vi "data_waypoint_ref.vi"() -> ()   [LabVIEW 2018] (continued)
{"X"=175318.28403795866, "Y"=530191.9350482963}, {"X"=175318.32304521388, "Y"=530191.9869078569}, {"X"=175318.36204793068, "Y"=530192.0384311461}, {"X"=175318.4005898055, "Y"=530192.0898758835}, {"X"=175318.43864458468, "Y"=530192.1416494689}, {"X"=175318.47640338843, "Y"=530192.1930820906}, {"X"=175318.51419378835, "Y"=530192.2441161796}, {"X"=175318.55208232062, "Y"=530192.2944862834}, {"X"=175318.58985834898, "Y"=530192.3451530531}, {"X"=175318.62736532633, "Y"=530192.3949971002}, {"X"=175318.66480275526, "Y"=530192.4440855398}, {"X"=175318.70216220792, "Y"=530192.4937657638}, {"X"=175318.74007465132, "Y"=530192.5435342542}, {"X"=175318.77838922056, "Y"=530192.5935956714}, {"X"=175318.81680214155, "Y"=530192.6436667865}, {"X"=175318.85473180335, "Y"=530192.6944685044}, {"X"=175318.893105015, "Y"=530192.7454908877}, {"X"=175318.93198027203, "Y"=530192.7964474163}, {"X"=175318.97074562093, "Y"=530192.847981396}, {"X"=175319.00950281188, "Y"=530192.8997518}, {"X"=175319.04856699263, "Y"=530192.9522948697}, {"X"=175319.08807038947, "Y"=530193.0047922492}, {"X"=175319.12802343152, "Y"=530193.0571762068}, {"X"=175319.16773230815, "Y"=530193.1099670911}, {"X"=175319.20749691897, "Y"=530193.1627333963}, {"X"=175319.24724586855, "Y"=530193.2155963047}, {"X"=175319.2868629425, "Y"=530193.2681954568}, {"X"=175319.32616219769, "Y"=530193.3205547077}, {"X"=175319.36573062692, "Y"=530193.3722783243}, {"X"=175319.4052265945, "Y"=530193.4237613154}, {"X"=175319.4445765745, "Y"=530193.4753002316}, {"X"=175319.48329824244, "Y"=530193.5267411147}, {"X"=175319.52202255937, "Y"=530193.5781808796}, {"X"=175319.56047417186, "Y"=530193.6296591858}, {"X"=175319.59880642896, "Y"=530193.6815151966}, {"X"=175319.6371569635, "Y"=530193.7326608438}, {"X"=175319.67575621096, "Y"=530193.7837424942}, {"X"=175319.71455607042, "Y"=530193.8343662901}, {"X"=175319.75346005248, "Y"=530193.8851551494}, {"X"=175319.7919885356, "Y"=530193.936569968}, {"X"=175319.83131689022, "Y"=530193.9879868631}, {"X"=175319.87087732382, "Y"=530194.0400046195}, {"X"=175319.91055584635, "Y"=530194.0927179083}, {"X"=175319.95018736875, "Y"=530194.1460129021}, {"X"=175319.99024830922, "Y"=530194.1992444766}, {"X"=175320.0305557881, "Y"=530194.2525741017}, {"X"=175320.0712095635, "Y"=530194.3052889514}, {"X"=175320.1119900287, "Y"=530194.3568103306}, {"X"=175320.15219124436, "Y"=530194.4083500657}, {"X"=175320.1921387411, "Y"=530194.458860601}, {"X"=175320.23155410215, "Y"=530194.5097467307}, {"X"=175320.2707313738, "Y"=530194.5609953767}, {"X"=175320.31042178915, "Y"=530194.6123379564}, {"X"=175320.35031262046, "Y"=530194.664057296}, {"X"=175320.3899530186, "Y"=530194.7158606148}, {"X"=175320.4297119804, "Y"=530194.767318418}, {"X"=175320.46997990887, "Y"=530194.8180544211}, {"X"=175320.51043847628, "Y"=530194.8688564525}, {"X"=175320.55115700723, "Y"=530194.9195034475}, {"X"=175320.5917810682, "Y"=530194.9702550462}, {"X"=175320.63193107033, "Y"=530195.0218526484}, {"X"=175320.67129892917, "Y"=530195.0737522215}, {"X"=175320.7100377912, "Y"=530195.1256225747}, {"X"=175320.74886255787, "Y"=530195.1768866911}, {"X"=175320.78829647583, "Y"=530195.2277594492}, {"X"=175320.82829674848, "Y"=530195.2781466381}, {"X"=175320.86779848064, "Y"=530195.3288871238}, {"X"=175320.90681250475, "Y"=530195.3794503614}, {"X"=175320.94602985482, "Y"=530195.429575715}, {"X"=175320.98480971038, "Y"=530195.4797301069}, {"X"=175321.02332181047, "Y"=530195.5292005048}, {"X"=175321.06128693797, "Y"=530195.57882124}, {"X"=175321.0995861466, "Y"=530195.6287894842}, {"X"=175321.1379527546, "Y"=530195.679084939}, {"X"=175321.17684378868, "Y"=530195.7290947222}, {"X"=175321.215752246, "Y"=530195.7787049029}, {"X"=175321.25457779068, "Y"=530195.8284340859}, {"X"=175321.2935347585, "Y"=530195.877373769}, {"X"=175321.33197582242, "Y"=530195.9267866664}, {"X"=175321.37019807613, "Y"=530195.9761924401}, {"X"=175321.40871088055, "Y"=530196.0256029064}, {"X"=175321.44677992928, "Y"=530196.0747216789}, {"X"=175321.48483888872, "Y"=530196.1231224035}, {"X"=175321.52257193413, "Y"=530196.1715429577}, {"X"=175321.56068217533, "Y"=530196.2202121164}, {"X"=175321.59924221472, "Y"=530196.2700208839}, {"X"=175321.63872254826, "Y"=530196.3210178126}, {"X"=175321.67865082875, "Y"=530196.3731266094}, {"X"=175321.71942213873, "Y"=530196.4266546473}, {"X"=175321.76037410757, "Y"=530196.4798691729}, {"X"=175321.80112038535, "Y"=530196.533019933}, {"X"=175321.8411714933, "Y"=530196.5856289156}, {"X"=175321.88069651256, "Y"=530196.6376612135}, {"X"=175321.9201304299, "Y"=530196.6885384173}, {"X"=175321.95949093453, "Y"=530196.7391528002}, {"X"=175321.99841810143, "Y"=530196.7900026427}, {"X"=175322.0373316636, "Y"=530196.8410456412}, {"X"=175322.0760458568, "Y"=530196.8926663568}, {"X"=175322.1152349461, "Y"=530196.9440259628}, {"X"=175322.1544901605, "Y"=530196.9952810451}, {"X"=175322.19440987587, "Y"=530197.0465907722}, {"X"=175322.23411659995, "Y"=530197.0980642746}, {"X"=175322.27372288413, "Y"=530197.1497212022}, {"X"=175322.31351665533, "Y"=530197.2012765786}, {"X"=175322.3533722951, "Y"=530197.2530859321}, {"X"=175322.39274468354, "Y"=530197.3041264676}, {"X"=175322.4312461575, "Y"=530197.3551040938}, {"X"=175322.4689193067, "Y"=530197.4054426665}, {"X"=175322.50720476272, "Y"=530197.454959244}, {"X"=175322.5459091693, "Y"=530197.5032659507}, {"X"=175322.58469188528, "Y"=530197.5513948477}, {"X"=175322.62243093, "Y"=530197.6003503415}, {"X"=175322.66002250477, "Y"=530197.64946276}, {"X"=175322.69777533837, "Y"=530197.6982894691}, {"X"=175322.7353187513, "Y"=530197.7469891632}, {"X"=175322.77224196383, "Y"=530197.7959381866}, {"X"=175322.80897855092, "Y"=530197.8452817602}, {"X"=175322.84632591892, "Y"=530197.8941851374}, {"X"=175322.88443607936, "Y"=530197.9437333102}, {"X"=175322.92386567718, "Y"=530197.9931510669}, {"X"=175322.96401642516, "Y"=530198.0432104138}, {"X"=175323.00403330493, "Y"=530198.0938306333}, {"X"=175323.04346028506, "Y"=530198.1450630171}, {"X"=175323.08229208103, "Y"=530198.196318245}, {"X"=175323.12123135975, "Y"=530198.2470748299}, {"X"=175323.15985042084, "Y"=530198.2982807423}, {"X"=175323.1988480503, "Y"=530198.3486997583}, {"X"=175323.23756583783, "Y"=530198.3991429065}, {"X"=175323.27665734818, "Y"=530198.4495583154}, {"X"=175323.31587152585, "Y"=530198.4992186585}, {"X"=175323.35479760286, "Y"=530198.5488043812}, {"X"=175323.39322686996, "Y"=530198.5981307524}, {"X"=175323.4315682364, "Y"=530198.6476860173}, {"X"=175323.46929583582, "Y"=530198.6969700654}, {"X"=175323.50722869192, "Y"=530198.7461702713}, {"X"=175323.5459397161, "Y"=530198.7946223526}, {"X"=175323.58439744834, "Y"=530198.8427899504}, {"X"=175323.62209566595, "Y"=530198.8917222602}, {"X"=175323.65877359055, "Y"=530198.9410005299}, {"X"=175323.69556244335, "Y"=530198.9900487311}, {"X"=175323.73411028614, "Y"=530199.0387354754}, {"X"=175323.77350876122, "Y"=530199.0881155926}, {"X"=175323.81290300708, "Y"=530199.1384646274}, {"X"=175323.85108638834, "Y"=530199.1891157913}, {"X"=175323.8888683214, "Y"=530199.2397037674}, {"X"=175323.92692682054, "Y"=530199.2885584359}, {"X"=175323.96485641086, "Y"=530199.3369540031}, {"X"=175324.00191990237, "Y"=530199.3851190561}, {"X"=175324.03842280654, "Y"=530199.4336209428}, {"X"=175324.07507156418, "Y"=530199.4829237162}, {"X"=175324.11335812218, "Y"=530199.5322183277}, {"X"=175324.15240360756, "Y"=530199.5817493182}, {"X"=175324.19127746008, "Y"=530199.6313518472}, {"X"=175324.2287002106, "Y"=530199.6817921636}, {"X"=175324.26553019526, "Y"=530199.7321742966}, {"X"=175324.30255214145, "Y"=530199.7815691971}, {"X"=175324.33997542586, "Y"=530199.8309895523}, {"X"=175324.3778948948, "Y"=530199.8801598336}, {"X"=175324.41578257747, "Y"=530199.929665387}, {"X"=175324.45303470409, "Y"=530199.9793193169}, {"X"=175324.49021220786, "Y"=530200.0288991062}, {"X"=175324.52719458667, "Y"=530200.0780943516}, {"X"=175324.56453317933, "Y"=530200.126432844}, {"X"=175324.6018519318, "Y"=530200.1752519632}, {"X"=175324.639619019, "Y"=530200.2247134796}, {"X"=175324.67763583743, "Y"=530200.2756559197}, {"X"=175324.71633669882, "Y"=530200.3275730183}, {"X"=175324.75549563722, "Y"=530200.3789316149}, {"X"=175324.79472103066, "Y"=530200.4299981245}, {"X"=175324.83290145468, "Y"=530200.4805516311}, {"X"=175324.8698345541, "Y"=530200.5307581061}, {"X"=175324.90571872293, "Y"=530200.5803106372}, {"X"=175324.94164630468, "Y"=530200.6292659377}, {"X"=175324.9781788097, "Y"=530200.6769974988}, {"X"=175325.01496359013, "Y"=530200.723770505}, {"X"=175325.05083836144, "Y"=530200.7713397482}, {"X"=175325.08665947133, "Y"=530200.8193353349}, {"X"=175325.12301564822, "Y"=530200.8679497532}, {"X"=175325.1597467984, "Y"=530200.9175597209}, {"X"=175325.1965801437, "Y"=530200.9678830262}, {"X"=175325.23368578497, "Y"=530201.0192288171}, {"X"=175325.27100025493, "Y"=530201.0708015133}, {"X"=175325.3086159226, "Y"=530201.1226851918}, {"X"=175325.3462306779, "Y"=530201.173658787}, {"X"=175325.38365508235, "Y"=530201.224064698}, {"X"=175325.42044835156, "Y"=530201.2740152087}, {"X"=175325.4568644001, "Y"=530201.3231078014}, {"X"=175325.49279309702, "Y"=530201.3721430111}, {"X"=175325.5287187662, "Y"=530201.4210528162}, {"X"=175325.56390410103, "Y"=530201.4709259429}, {"X"=175325.59903368057, "Y"=530201.5214163167}, {"X"=175325.63438651664, "Y"=530201.5719193501}, {"X"=175325.67106088204, "Y"=530201.6224007264}, {"X"=175325.70852292405, "Y"=530201.672954138}, {"X"=175325.74600077514, "Y"=530201.724963639}, {"X"=175325.78311414344, "Y"=530201.7780296917}, {"X"=175325.8204649508, "Y"=530201.8323125597}, {"X"=175325.85848104864, "Y"=530201.8872194239}, {"X"=175325.89734364732, "Y"=530201.9414190304}, {"X"=175325.93574889482, "Y"=530201.9949218861}, {"X"=175325.9731610076, "Y"=530202.0477684161}, {"X"=175326.00978406958, "Y"=530202.100076773}, {"X"=175326.0468937723, "Y"=530202.1507011494}, {"X"=175326.083703109, "Y"=530202.2006971186}, {"X"=175326.11978964065, "Y"=530202.2500903491}, {"X"=175326.15506203403, "Y"=530202.2991508055}, {"X"=175326.18999830802, "Y"=530202.3477727488}, {"X"=175326.2249742177, "Y"=530202.3954179}, {"X"=175326.26010835878, "Y"=530202.4426541552}, {"X"=175326.2947142973, "Y"=530202.4894968602}, {"X"=175326.32881687392, "Y"=530202.536559692}, {"X"=175326.36266935102, "Y"=530202.5844190321}, {"X"=175326.39759400964, "Y"=530202.6330077152}, {"X"=175326.43383685724, "Y"=530202.683445973}, {"X"=175326.47190138185, "Y"=530202.7349532002}, {"X"=175326.51121043155, "Y"=530202.7876609504}, {"X"=175326.55136520957, "Y"=530202.8415015922}, {"X"=175326.59171968058, "Y"=530202.8960752623}, {"X"=175326.6321905429, "Y"=530202.9510703352}, {"X"=175326.6722261586, "Y"=530203.0062542596}, {"X"=175326.71219305095, "Y"=530203.0615638003}, {"X"=175326.75209383233, "Y"=530203.116381868}, {"X"=175326.7917454435, "Y"=530203.1711107733}, {"X"=175326.83161576497, "Y"=530203.2246126398}, {"X"=175326.87189651153, "Y"=530203.2770178622}, {"X"=175326.91170643645, "Y"=530203.3286631126}, {"X"=175326.9508110747, "Y"=530203.3796411991}, {"X"=175326.98866926372, "Y"=530203.4302678084}, {"X"=175327.02652639092, "Y"=530203.4799343928}, {"X"=175327.06383915478, "Y"=530203.5291353314}, {"X"=175327.1012313738, "Y"=530203.5773460448}, {"X"=175327.13767728163, "Y"=530203.62515778}, {"X"=175327.1733785629, "Y"=530203.6724767144}, {"X"=175327.20888498292, "Y"=530203.7192002304}, {"X"=175327.24457231665, "Y"=530203.7662961268}, {"X"=175327.28073190898, "Y"=530203.8137380134}, {"X"=175327.31828937924, "Y"=530203.8621169378}, {"X"=175327.3568467017, "Y"=530203.9113286342}, {"X"=175327.39573231337, "Y"=530203.9613273641}, {"X"=175327.4348463128, "Y"=530204.0118770179}, {"X"=175327.4746820218, "Y"=530204.0623568422}, {"X"=175327.51439785375, "Y"=530204.1136372288}, {"X"=175327.55409277766, "Y"=530204.1650364326}, {"X"=175327.59377426372, "Y"=530204.2166853956}, {"X"=175327.63384299536, "Y"=530204.2683875972}, {"X"=175327.67389632692, "Y"=530204.3193728758}, {"X"=175327.71366109003, "Y"=530204.3698262745}, {"X"=175327.75270769326, "Y"=530204.419750169}, {"X"=175327.7914221135, "Y"=530204.4690701697}, {"X"=175327.82960123813, "Y"=530204.517694761}, {"X"=175327.86709288435, "Y"=530204.5662825343}, {"X"=175327.9041485433, "Y"=530204.6145086712}, {"X"=175327.94210074993, "Y"=530204.6615801282}, {"X"=175327.9798551974, "Y"=530204.7091738019}, {"X"=175328.0173480477, "Y"=530204.7569702436}, {"X"=175328.05459147744, "Y"=530204.8057918225}, {"X"=175328.09215344326, "Y"=530204.8553971305}, {"X"=175328.13028118102, "Y"=530204.9055201834}, {"X"=175328.16931487413, "Y"=530204.9561744055}, {"X"=175328.20865300385, "Y"=530205.0073360448}, {"X"=175328.24843108968, "Y"=530205.0590047016}, {"X"=175328.28835976106, "Y"=530205.110072481}, {"X"=175328.3279304532, "Y"=530205.1607994803}, {"X"=175328.36635310898, "Y"=530205.2115076702}, {"X"=175328.4048222024, "Y"=530205.2614421498}, {"X"=175328.44354148043, "Y"=530205.3115112955}, {"X"=175328.48294085654, "Y"=530205.3621167176}, {"X"=175328.52195241617, "Y"=530205.4139774231}, {"X"=175328.56165370328, "Y"=530205.4657362077}, {"X"=175328.60110805032, "Y"=530205.5175612008}, {"X"=175328.6405652865, "Y"=530205.568864554}, {"X"=175328.6796272788, "Y"=530205.619805039}, {"X"=175328.71811733616, "Y"=530205.670242225}, {"X"=175328.75615469483, "Y"=530205.7197573447}, {"X"=175328.79388382484, "Y"=530205.7689803721}, {"X"=175328.83173539452, "Y"=530205.8179721874}, {"X"=175328.86998914456, "Y"=530205.8666753601}, {"X"=175328.90845591988, "Y"=530205.9152258562}, {"X"=175328.94701416916, "Y"=530205.9638582114}, {"X"=175328.98495470296, "Y"=530206.0135811617}, {"X"=175329.02283770952, "Y"=530206.063320929}, {"X"=175329.061211757, "Y"=530206.1137684488}, {"X"=175329.1004535877, "Y"=530206.1644198417}, {"X"=175329.13965264565, "Y"=530206.215584116}, {"X"=175329.17943126732, "Y"=530206.2665369152}, {"X"=175329.21919262805, "Y"=530206.3173443769}, {"X"=175329.25909633044, "Y"=530206.3683600716}, {"X"=175329.29923168753, "Y"=530206.4189333583}, {"X"=175329.33950991664, "Y"=530206.4692942395}, {"X"=175329.37883474256, "Y"=530206.5198543807}, {"X"=175329.4174794207, "Y"=530206.5710624671}, {"X"=175329.45618161428, "Y"=530206.6222492951}, {"X"=175329.49601390955, "Y"=530206.6721808698}, {"X"=175329.53568236195, "Y"=530206.7218221434}, {"X"=175329.57487133163, "Y"=530206.7710708327}, {"X"=175329.61317725817, "Y"=530206.8203476531}, {"X"=175329.65166145592, "Y"=530206.868802654}, {"X"=175329.69034324563, "Y"=530206.9169784943}, {"X"=175329.72884437937, "Y"=530206.9657686227}, {"X"=175329.76712680032, "Y"=530207.0151864667}, {"X"=175329.80580621227, "Y"=530207.0652579557}, {"X"=175329.84515547164, "Y"=530207.1153951712}, {"X"=175329.88507176263, "Y"=530207.1655773262}, {"X"=175329.92491169384, "Y"=530207.2159972164}, {"X"=175329.96473889175, "Y"=530207.2666047115}, {"X"=175330.0045233484, "Y"=530207.3177372969}, {"X"=175330.04477562633, "Y"=530207.3689128957}, {"X"=175330.08507576596, "Y"=530207.4206987759}, {"X"=175330.12605519747, "Y"=530207.4715492621}, {"X"=175330.16637356245, "Y"=530207.5226070208}, {"X"=175330.20511206114, "Y"=530207.5740934082}, {"X"=175330.24271986936, "Y"=530207.6257351815}, {"X"=175330.2810642061, "Y"=530207.6763248568}, {"X"=175330.31986330473, "Y"=530207.7258344068}, {"X"=175330.35768402094, "Y"=530207.775783018}, {"X"=175330.39437893714, "Y"=530207.8254430583}, {"X"=175330.4313906394, "Y"=530207.874092192}, {"X"=175330.46888017948, "Y"=530207.921375898}, {"X"=175330.50616064473, "Y"=530207.9677490287}, {"X"=175330.5426012657, "Y"=530208.0146817855}, {"X"=175330.57887375378, "Y"=530208.0619724141}, {"X"=175330.61506270058, "Y"=530208.1103698179}, {"X"=175330.65235307286, "Y"=530208.1595009197}, {"X"=175330.6898371192, "Y"=530208.2097268798}, {"X"=175330.72784761153, "Y"=530208.2603519466}, {"X"=175330.7657841934, "Y"=530208.3108440499}, {"X"=175330.80350983172, "Y"=530208.361594262}, {"X"=175330.84116910724, "Y"=530208.4123679763}, {"X"=175330.8800341823, "Y"=530208.4632258139}, {"X"=175330.91904552278, "Y"=530208.5144217251}, {"X"=175330.95728834765, "Y"=530208.5660349927}, {"X"=175330.99433718255, "Y"=530208.6182655349}, {"X"=175331.0318488113, "Y"=530208.6688343638}, {"X"=175331.06905319763, "Y"=530208.7185461762}, {"X"=175331.10566655878, "Y"=530208.7675871584}, {"X"=175331.14137250715, "Y"=530208.8168039559}, {"X"=175331.17715414436, "Y"=530208.8661548237}, {"X"=175331.21332360696, "Y"=530208.9154568233}, {"X"=175331.25029619085, "Y"=530208.9649606678}, {"X"=175331.2873574178, "Y"=530209.0144875587}, {"X"=175331.32414960433, "Y"=530209.0643948126}, {"X"=175331.36084215975, "Y"=530209.114159192}, {"X"=175331.3975425129, "Y"=530209.1638647242}, {"X"=175331.43446336297, "Y"=530209.2144497242}, {"X"=175331.47308668031, "Y"=530209.2647300402}, {"X"=175331.51153533268, "Y"=530209.315855475}, {"X"=175331.54889317372, "Y"=530209.3674425003}, {"X"=175331.5855494454, "Y"=530209.4196220397}, {"X"=175331.62295978758, "Y"=530209.4709902672}, {"X"=175331.66061267612, "Y"=530209.5217040731}, {"X"=175331.69814321943, "Y"=530209.5723827237}, {"X"=175331.73536540987, "Y"=530209.6233275409}, {"X"=175331.77258882776, "Y"=530209.6746885533}, {"X"=175331.80997591818, "Y"=530209.7262832607}, {"X"=175331.8481199299, "Y"=530209.7774340136}, {"X"=175331.88623244286, "Y"=530209.8287158216}, {"X"=175331.9241847472, "Y"=530209.8794387324}, {"X"=175331.96143662307, "Y"=530209.9299384085}, {"X"=175331.99790744064, "Y"=530209.9799065489}, {"X"=175332.03363035072, "Y"=530210.0303718917}, {"X"=175332.07052518567, "Y"=530210.0802477727}, {"X"=175332.10833857156, "Y"=530210.1304217139}, {"X"=175332.14653489395, "Y"=530210.1818897336}, {"X"=175332.1846024039, "Y"=530210.2341328121}, {"X"=175332.22300738035, "Y"=530210.2869697822}, {"X"=175332.2621362657, "Y"=530210.339582644}, {"X"=175332.30199405577, "Y"=530210.3918626182}, {"X"=175332.34141600237, "Y"=530210.4441305593}, {"X"=175332.38041804795, "Y"=530210.4963853122}, {"X"=175332.4185211116, "Y"=530210.5486704636}, {"X"=175332.45682697443, "Y"=530210.5997386106}, {"X"=175332.49514308042, "Y"=530210.6506768743}, {"X"=175332.53412157384, "Y"=530210.7006542655}, {"X"=175332.57272378285, "Y"=530210.7512909137}, {"X"=175332.61101197888, "Y"=530210.8029773051}, {"X"=175332.64921056182, "Y"=530210.8558148851}, {"X"=175332.68851538797, "Y"=530210.9095182215}, {"X"=175332.72771294997, "Y"=530210.9640942254}, {"X"=175332.76750234602, "Y"=530211.0190136484}, {"X"=175332.80752506072, "Y"=530211.0731554804}, {"X"=175332.84765670967, "Y"=530211.1269895624}, {"X"=175332.88795444716, "Y"=530211.1803758806}, {"X"=175332.92839109115, "Y"=530211.234007068}, {"X"=175332.96848531367, "Y"=530211.2886669956}, {"X"=175333.0089040344, "Y"=530211.3437299544}, {"X"=175333.0491415058, "Y"=530211.3989066537}, {"X"=175333.08910233053, "Y"=530211.4539887221}, {"X"=175333.1285585995, "Y"=530211.5088869324}, {"X"=175333.16815412405, "Y"=530211.5626471259}, {"X"=175333.20753422027, "Y"=530211.6163446938}, {"X"=175333.2473421582, "Y"=530211.6697457767}, {"X"=175333.28705198405, "Y"=530211.724119386}, {"X"=175333.3265540142, "Y"=530211.779216127}, {"X"=175333.3660775373, "Y"=530211.8349931492}, {"X"=175333.40622949848, "Y"=530211.8900102822}, {"X"=175333.44650034822, "Y"=530211.9444932247}, {"X"=175333.48723672854, "Y"=530211.9985430562}, {"X"=175333.52736064664, "Y"=530212.0530630564}, {"X"=175333.56740341955, "Y"=530212.1080017141}, {"X"=175333.6077093309, "Y"=530212.1626599086}, {"X"=175333.64857199727, "Y"=530212.2168813988}, {"X"=175333.68922026566, "Y"=530212.2707905404}, {"X"=175333.72890749428, "Y"=530212.3247113958}, {"X"=175333.76778450757, "Y"=530212.3784270975}, {"X"=175333.80736747183, "Y"=530212.4321351693}, {"X"=175333.84828877196, "Y"=530212.4858159842}, {"X"=175333.88984022452, "Y"=530212.539917797}, {"X"=175333.93109660895, "Y"=530212.5948872815}, {"X"=175333.97284515807, "Y"=530212.6497432184}, {"X"=175334.0142686215, "Y"=530212.7046001133}, {"X"=175334.05544437704, "Y"=530212.7586608616}, {"X"=175334.0959890387, "Y"=530212.8128810698}, {"X"=175334.13627522383, "Y"=530212.8671608662}, {"X"=175334.17651603464, "Y"=530212.9222742985}, {"X"=175334.2177644458, "Y"=530212.9772438075}, {"X"=175334.25957639978, "Y"=530213.0322760266}, {"X"=175334.30213095952, "Y"=530213.0865147257}, {"X"=175334.34455506905, "Y"=530213.1406738986}, {"X"=175334.38594238626, "Y"=530213.195288953}, {"X"=175334.42704816477, "Y"=530213.2499525625}, {"X"=175334.46824282644, "Y"=530213.3047191269}, {"X"=175334.50961381703, "Y"=530213.3595051488}, {"X"=175334.55108627415, "Y"=530213.4141565791}, {"X"=175334.59266786097, "Y"=530213.4679675244}, {"X"=175334.63399788298, "Y"=530213.5211776675}, {"X"=175334.6750819692, "Y"=530213.573293105}, {"X"=175334.71570326976, "Y"=530213.6252711763}, {"X"=175334.75589895574, "Y"=530213.6780007676}, {"X"=175334.79658751158, "Y"=530213.7311584209}, {"X"=175334.83711118187, "Y"=530213.7854730334}, {"X"=175334.87751620755, "Y"=530213.8401054167}, {"X"=175334.9179042401, "Y"=530213.894081924}, {"X"=175334.95911596806, "Y"=530213.9465288344}, {"X"=175334.99991220928, "Y"=530213.9986573323}, {"X"=175335.04026648914, "Y"=530214.050201127}, {"X"=175335.08012203232, "Y"=530214.1026320615}, {"X"=175335.12058568108, "Y"=530214.1555184657}, {"X"=175335.16164489972, "Y"=530214.2088137578}, {"X"=175335.2026623043, "Y"=530214.2629493396}, {"X"=175335.24292566493, "Y"=530214.317904002}, {"X"=175335.2838600399, "Y"=530214.3724194007}, {"X"=175335.32589039847, "Y"=530214.4264254693}, {"X"=175335.36913003057, "Y"=530214.4801915719}, {"X"=175335.4125249086, "Y"=530214.5343367882}, {"X"=175335.45555095756, "Y"=530214.5889669928}, {"X"=175335.49830331592, "Y"=530214.6433027806}, {"X"=175335.54073540578, "Y"=530214.6974685959}, {"X"=175335.58196774634, "Y"=530214.7521007617}, {"X"=175335.62354322325, "Y"=530214.8059483555}, {"X"=175335.66565024323, "Y"=530214.8586179304}, {"X"=175335.70747625933, "Y"=530214.9106157594}, {"X"=175335.7480881228, "Y"=530214.963002292}, {"X"=175335.7885573149, "Y"=530215.0144669515}, {"X"=175335.82880391076, "Y"=530215.0658434787}, {"X"=175335.86905572907, "Y"=530215.1162866012}, {"X"=175335.909482951, "Y"=530215.1667380838}, {"X"=175335.95024341732, "Y"=530215.2175526178}, {"X"=175335.9909282017, "Y"=530215.2700366036}, {"X"=175336.03225353497, "Y"=530215.3231646375}, {"X"=175336.0742294917, "Y"=530215.3758479197}, {"X"=175336.1162228887, "Y"=530215.4281371495}, {"X"=175336.15780792251, "Y"=530215.480420926}, {"X"=175336.198753351, "Y"=530215.5338830402}, {"X"=175336.2400447598, "Y"=530215.5884240265}, {"X"=175336.28280096015, "Y"=530215.6431649067}, {"X"=175336.32627274963, "Y"=530215.697862611}, {"X"=175336.3695396637, "Y"=530215.7518728063}, {"X"=175336.41189431006, "Y"=530215.8050133444}, {"X"=175336.4530581296, "Y"=530215.857140764}, {"X"=175336.4923324384, "Y"=530215.9083226097}, {"X"=175336.53024073623, "Y"=530215.9582587824}, {"X"=175336.56758054454, "Y"=530216.0079569012}, {"X"=175336.60624975662, "Y"=530216.0567010613}, {"X"=175336.64522401133, "Y"=530216.1052567544}, {"X"=175336.68329837156, "Y"=530216.1538350807}, {"X"=175336.72042406868, "Y"=530216.2021165418}, {"X"=175336.75789178454, "Y"=530216.2498342964}, {"X"=175336.79601195845, "Y"=530216.2977277045}, {"X"=175336.83490120104, "Y"=530216.3474945049}, {"X"=175336.8747391946, "Y"=530216.3987878956}, {"X"=175336.9155644031, "Y"=530216.4511349584}, {"X"=175336.9565872925, "Y"=530216.5038343738}, {"X"=175336.99702923294, "Y"=530216.5562757964}, {"X"=175337.03653662247, "Y"=530216.608701107}, {"X"=175337.07562676386, "Y"=530216.6599112444}, {"X"=175337.11431845836, "Y"=530216.7105731766}, {"X"=175337.15316399393, "Y"=530216.7608384356}, {"X"=175337.19213873718, "Y"=530216.8122653349}, {"X"=175337.232309873, "Y"=530216.8641903627}, {"X"=175337.27302243776, "Y"=530216.9167896998}, {"X"=175337.31390302093, "Y"=530216.9698935254}, {"X"=175337.3542175054, "Y"=530217.0235705986}, {"X"=175337.39383505605, "Y"=530217.0782097556}, {"X"=175337.43345427106, "Y"=530217.1331130541}, {"X"=175337.4731671136, "Y"=530217.1885266124}, {"X"=175337.51269825146, "Y"=530217.2435999815}, {"X"=175337.55194491986, "Y"=530217.2977274793}, {"X"=175337.59038441366, "Y"=530217.3505776902}, {"X"=175337.62842923752, "Y"=530217.40235916}, {"X"=175337.6661001939, "Y"=530217.4535179922}, {"X"=175337.70416076016, "Y"=530217.5037300759}, {"X"=175337.7420038972, "Y"=530217.5544022826}, {"X"=175337.7794317696, "Y"=530217.6051323175}, {"X"=175337.81701866104, "Y"=530217.6563202547}, {"X"=175337.8544032769, "Y"=530217.708001567}, {"X"=175337.8925377935, "Y"=530217.7595608027}, {"X"=175337.93128742423, "Y"=530217.8109495258}, {"X"=175337.9695507337, "Y"=530217.8629301275}, {"X"=175338.0082516581, "Y"=530217.9152235296}, {"X"=175338.04761985684, "Y"=530217.967611521}, {"X"=175338.08728319546, "Y"=530218.0209597816}, {"X"=175338.1271335317, "Y"=530218.0749423284}, {"X"=175338.16702309356, "Y"=530218.1290091096}, {"X"=175338.20661768012, "Y"=530218.1830734315}, {"X"=175338.2461740608, "Y"=530218.2367982493}, {"X"=175338.28507050654, "Y"=530218.2905139152}, {"X"=175338.32402685797, "Y"=530218.3435179845}, {"X"=175338.3628983841, "Y"=530218.3962936742}, {"X"=175338.40248170623, "Y"=530218.4477409829}, {"X"=175338.44199884526, "Y"=530218.4989731741}, {"X"=175338.4810465143, "Y"=530218.5499037582}, {"X"=175338.51934318643, "Y"=530218.600885391}, {"X"=175338.55710943416, "Y"=530218.6522204147}, {"X"=175338.5948762553, "Y"=530218.7037507715}, {"X"=175338.6338252904, "Y"=530218.7548769822}, {"X"=175338.6739002579, "Y"=530218.8060364973}, {"X"=175338.71384854216, "Y"=530218.8583928163}, {"X"=175338.753222827, "Y"=530218.9113457106}, {"X"=175338.792356318, "Y"=530218.9646467023}, {"X"=175338.8311580059, "Y"=530219.01837153}, {"X"=175338.87071642242, "Y"=530219.0715880294}, {"X"=175338.91075334582, "Y"=530219.1254668134}, {"X"=175338.95190623117, "Y"=530219.1793034604}, {"X"=175338.99320496703, "Y"=530219.2336380056}, {"X"=175339.03450596903, "Y"=530219.2878393602}, {"X"=175339.07593600373, "Y"=530219.3419426669}, {"X"=175339.1173234146, "Y"=530219.3954090409}, {"X"=175339.15756587937, "Y"=530219.4490019855}, {"X"=175339.196607049, "Y"=530219.5022366615}, {"X"=175339.23502417348, "Y"=530219.5550181346}, {"X"=175339.27417272714, "Y"=530219.6071215451}, {"X"=175339.31415161595, "Y"=530219.6584433867}, {"X"=175339.35397403524, "Y"=530219.7095736838}, {"X"=175339.3928394618, "Y"=530219.7608854916}, {"X"=175339.43153280398, "Y"=530219.8121156775}, {"X"=175339.4711378264, "Y"=530219.8631167639}, {"X"=175339.5113195704, "Y"=530219.9153447627}, {"X"=175339.5514793716, "Y"=530219.968542844}, {"X"=175339.59169131416, "Y"=530220.0223001395}, {"X"=175339.63130955625, "Y"=530220.077183476}, {"X"=175339.6713096225, "Y"=530220.1317837801}, {"X"=175339.71162398445, "Y"=530220.1860302234}, {"X"=175339.75238126508, "Y"=530220.2396849147}, {"X"=175339.79291413393, "Y"=530220.2938363759}, {"X"=175339.8341795131, "Y"=530220.3476771363}, {"X"=175339.87538622756, "Y"=530220.4017489201}, {"X"=175339.91570330068, "Y"=530220.4557134501}, {"X"=175339.95501255686, "Y"=530220.5094489943}, {"X"=175339.99378179503, "Y"=530220.5623881428}, {"X"=175340.032220397, "Y"=530220.614045269}, {"X"=175340.0706813909, "Y"=530220.6642850373}, {"X"=175340.1095277134, "Y"=530220.7136280148}, {"X"=175340.1483784491, "Y"=530220.7632662015}, {"X"=175340.1866975091, "Y"=530220.8131345876}, {"X"=175340.22491300027, "Y"=530220.8627269252}, {"X"=175340.26314188118, "Y"=530220.9126532906}, {"X"=175340.30124549245, "Y"=530220.9624546103}, {"X"=175340.3389347308, "Y"=530221.0126145277}, {"X"=175340.3772862895, "Y"=530221.0623907007}, {"X"=175340.41577064258, "Y"=530221.1127436082}, {"X"=175340.45473172294, "Y"=530221.1634558148}, {"X"=175340.49399150687, "Y"=530221.2139340698}, {"X"=175340.53319028806, "Y"=530221.2641516883}, {"X"=175340.57132779274, "Y"=530221.3143324822}, {"X"=175340.60874069866, "Y"=530221.3645043136}, {"X"=175340.64630832113, "Y"=530221.4133749353}, {"X"=175340.68330462027, "Y"=530221.4616479168}, {"X"=175340.7200604363, "Y"=530221.5097728887}, {"X"=175340.7568127796, "Y"=530221.5576215149}, {"X"=175340.79352235922, "Y"=530221.6056866894}, {"X"=175340.83133687428, "Y"=530221.6532746962}, {"X"=175340.86972653927, "Y"=530221.701257226}, {"X"=175340.9080893437, "Y"=530221.7497437114}, {"X"=175340.9458108464, "Y"=530221.7991321841}, {"X"=175340.98414187023, "Y"=530221.8497574623}, {"X"=175341.02349582317, "Y"=530221.9009324348}, {"X"=175341.06375182403, "Y"=530221.9531158272}, {"X"=175341.1044829561, "Y"=530222.005719567}, {"X"=175341.14595957266, "Y"=530222.0579060195}, {"X"=175341.1872804957, "Y"=530222.1101617429}, {"X"=175341.2283713614, "Y"=530222.1619009508}, {"X"=175341.26824615517, "Y"=530222.213376271}, {"X"=175341.3077069612, "Y"=530222.2638406174}, {"X"=175341.3464592256, "Y"=530222.3143336911}, {"X"=175341.38514233282, "Y"=530222.3636039045}, {"X"=175341.42348113446, "Y"=530222.4123623798}, {"X"=175341.4619506573, "Y"=530222.4606942837}, {"X"=175341.500862789, "Y"=530222.5080282264}, {"X"=175341.53989545174, "Y"=530222.5556858942}, {"X"=175341.57855971582, "Y"=530222.6045743736}, {"X"=175341.61733350207, "Y"=530222.6548576218}, {"X"=175341.65613315726, "Y"=530222.7061030421}, {"X"=175341.69501567204, "Y"=530222.7578132504}, {"X"=175341.7343073941, "Y"=530222.8095144829}, {"X"=175341.77426430586, "Y"=530222.8600028963}, {"X"=175341.81392813384, "Y"=530222.9102291381}, {"X"=175341.85343851932, "Y"=530222.9594858147}, {"X"=175341.89225202618, "Y"=530223.0088222381}, {"X"=175341.93099129558, "Y"=530223.0579147108}, {"X"=175341.96965254052, "Y"=530223.1075823216}, {"X"=175342.0079390977, "Y"=530223.1578514714}, {"X"=175342.04531629087, "Y"=530223.208234289}, {"X"=175342.0823620307, "Y"=530223.2582584881}, {"X"=175342.12036757922, "Y"=530223.3069524673}, {"X"=175342.15868380744, "Y"=530223.3555689492}, {"X"=175342.19669862968, "Y"=530223.4053061692}, {"X"=175342.235050533, "Y"=530223.455206654}, {"X"=175342.2738534825, "Y"=530223.5063710476}, {"X"=175342.31314116152, "Y"=530223.5582054758}, {"X"=175342.35286638304, "Y"=530223.6106301709}, {"X"=175342.39277461008, "Y"=530223.6626336892}, {"X"=175342.43220801378, "Y"=530223.7146241793}, {"X"=175342.47159401196, "Y"=530223.7661575475}, {"X"=175342.51108410227, "Y"=530223.8175463284}, {"X"=175342.55094774097, "Y"=530223.869450092}, {"X"=175342.5912302505, "Y"=530223.9216189857}, {"X"=175342.63127412286, "Y"=530223.9742658229}, {"X"=175342.67080800404, "Y"=530224.0272881878}, {"X"=175342.71031867288, "Y"=530224.0796480348}, {"X"=175342.74951846778, "Y"=530224.1317202356}, {"X"=175342.78877232302, "Y"=530224.1828999498}, {"X"=175342.82772654106, "Y"=530224.2342991909}, {"X"=175342.86694903608, "Y"=530224.2847575897}, {"X"=175342.90560732182, "Y"=530224.3358291847}, {"X"=175342.94384633898, "Y"=530224.3871017921}, {"X"=175342.9820561291, "Y"=530224.4380759329}, {"X"=175343.02040845525, "Y"=530224.4887244644}, {"X"=175343.05860425235, "Y"=530224.539158146}, {"X"=175343.09711823752, "Y"=530224.5899571424}, {"X"=175343.1359562095, "Y"=530224.6415875782}, {"X"=175343.17549843973, "Y"=530224.6935377966}, {"X"=175343.21551242692, "Y"=530224.7456653102}, {"X"=175343.25560978387, "Y"=530224.7972276604}, {"X"=175343.29504013137, "Y"=530224.849386863}, {"X"=175343.3341498303, "Y"=530224.9012462393}, {"X"=175343.37274251977, "Y"=530224.9538052416}, {"X"=175343.41201237464, "Y"=530225.0068095207}, {"X"=175343.451815017, "Y"=530225.0602606118}, {"X"=175343.49195184934, "Y"=530225.1131957419}, {"X"=175343.53112082684, "Y"=530225.1662347257}, {"X"=175343.56961757506, "Y"=530225.219001554}, {"X"=175343.6080597585, "Y"=530225.2706864333}, {"X"=175343.64636462432, "Y"=530225.3217635131}, {"X"=175343.68403406208, "Y"=530225.3727314826}, {"X"=175343.7218600944, "Y"=530225.4236357275}, {"X"=175343.7595005975, "Y"=530225.4756059833}, {"X"=175343.79804115012, "Y"=530225.5279087643}, {"X"=175343.8375512105, "Y"=530225.5809689405}, {"X"=175343.87768913654, "Y"=530225.634275872}, {"X"=175343.917179842, "Y"=530225.6888821401}, {"X"=175343.95703650004, "Y"=530225.7435317221}, {"X"=175343.99699233004, "Y"=530225.7993696701}, {"X"=175344.0379195635, "Y"=530225.8560071833}, {"X"=175344.07954486008, "Y"=530225.9129678269}, {"X"=175344.1215070291, "Y"=530225.9700218146}, {"X"=175344.16306955542, "Y"=530226.0270237095}, {"X"=175344.20444305483, "Y"=530226.0836044145}, {"X"=175344.2454281164, "Y"=530226.140028664}, {"X"=175344.2863313288, "Y"=530226.1963310726}, {"X"=175344.32693259235, "Y"=530226.2520683417}, {"X"=175344.3668732474, "Y"=530226.3081693741}, {"X"=175344.40610914843, "Y"=530226.3646831337}, {"X"=175344.44565920217, "Y"=530226.4204934239}, {"X"=175344.48556397823, "Y"=530226.4755424161}, {"X"=175344.52579878274, "Y"=530226.5292641538}, {"X"=175344.56470778922, "Y"=530226.5830608321}, {"X"=175344.60305079306, "Y"=530226.6368625081}, {"X"=175344.64138657736, "Y"=530226.6909194754}, {"X"=175344.6803523717, "Y"=530226.7450500538}, {"X"=175344.7192578378, "Y"=530226.8000498302}, {"X"=175344.75917082647, "Y"=530226.8551809292}, {"X"=175344.79916464357, "Y"=530226.9115892368}, {"X"=175344.83981818473, "Y"=530226.9691365355}, {"X"=175344.88087487346, "Y"=530227.0279256878}, {"X"=175344.92272513863, "Y"=530227.0869855267}, {"X"=175344.96484817393, "Y"=530227.1460290228}, {"X"=175345.00702341314, "Y"=530227.2047527262}, {"X"=175345.04837276042, "Y"=530227.2636608795}, {"X"=175345.08951531787, "Y"=530227.322132361}, {"X"=175345.13091765594, "Y"=530227.3797862194}, {"X"=175345.17261180005, "Y"=530227.4369697464}, {"X"=175345.2138841165, "Y"=530227.4943875886}, {"X"=175345.25474182, "Y"=530227.5523837806}, {"X"=175345.2953319248, "Y"=530227.6103496855}, {"X"=175345.33608077082, "Y"=530227.6677768407}, {"X"=175345.3767031518, "Y"=530227.7246727465}, {"X"=175345.41711203125, "Y"=530227.7815592935}, {"X"=175345.45734774778, "Y"=530227.8385984013}, {"X"=175345.49814907316, "Y"=530227.8961008744}, {"X"=175345.53987397553, "Y"=530227.9535040656}, {"X"=175345.58270584818, "Y"=530228.0105188708}, {"X"=175345.62524984934, "Y"=530228.0681371794}, {"X"=175345.66747818922, "Y"=530228.1265477482}, {"X"=175345.70959393718, "Y"=530228.1852261261}, {"X"=175345.7526580195, "Y"=530228.2440892733}, {"X"=175345.79605483665, "Y"=530228.3031445545}, {"X"=175345.8397833751, "Y"=530228.362049028}, {"X"=175345.8829142793, "Y"=530228.4219463692}, {"X"=175345.92626609065, "Y"=530228.4816599311}, {"X"=175345.96973678764, "Y"=530228.5405385285}, {"X"=175346.0128790672, "Y"=530228.5985868099}, {"X"=175346.05557086875, "Y"=530228.6564643917}, {"X"=175346.09855932498, "Y"=530228.7140148013}, {"X"=175346.14169494555, "Y"=530228.7716069507}, {"X"=175346.18538720495, "Y"=530228.8284227776}, {"X"=175346.2289090404, "Y"=530228.8851192427}, {"X"=175346.27231195508, "Y"=530228.9411379342}, {"X"=175346.31467855422, "Y"=530228.9977745438}, {"X"=175346.3565197893, "Y"=530229.0540797464}, {"X"=175346.398209656, "Y"=530229.1098182551}, {"X"=175346.44036334916, "Y"=530229.1648461967}, {"X"=175346.48222626268, "Y"=530229.2206929632}, {"X"=175346.5240881895, "Y"=530229.2768060985}, {"X"=175346.56605635298, "Y"=530229.3332008257}, {"X"=175346.60913138627, "Y"=530229.3894735328}, {"X"=175346.65260054462, "Y"=530229.4460303147}, {"X"=175346.6961474528, "Y"=530229.5031207076}, {"X"=175346.73861139643, "Y"=530229.5606304918}, {"X"=175346.78057418144, "Y"=530229.6182061245}, {"X"=175346.8221392308, "Y"=530229.6754743905}, {"X"=175346.8638107502, "Y"=530229.7325026138}, {"X"=175346.90517967637, "Y"=530229.789648263}, {"X"=175346.94734387382, "Y"=530229.8467382959}, {"X"=175346.99017519283, "Y"=530229.9032714318}, {"X"=175347.03319368736, "Y"=530229.9604987887}, {"X"=175347.07558367634, "Y"=530230.0181630625}, {"X"=175347.1179610232, "Y"=530230.0760460165}, {"X"=175347.16041506414, "Y"=530230.1341029915}, {"X"=175347.20272800326, "Y"=530230.1926742499}, {"X"=175347.24512683423, "Y"=530230.2515349273}, {"X"=175347.2874182252, "Y"=530230.3109086764}, {"X"=175347.3299874161, "Y"=530230.3695679661}, {"X"=175347.37305761402, "Y"=530230.4275088108}, {"X"=175347.41586943413, "Y"=530230.4849409934}, {"X"=175347.45826517747, "Y"=530230.5418549861}, {"X"=175347.50003243302, "Y"=530230.5983091341}, {"X"=175347.54152667837, "Y"=530230.6550004845}, {"X"=175347.5828384125, "Y"=530230.7116779468}, {"X"=175347.62513317316, "Y"=530230.7676899249}, {"X"=175347.66725613666, "Y"=530230.8237168362}, {"X"=175347.70895552073, "Y"=530230.8796850655}, {"X"=175347.75047259853, "Y"=530230.936010097}, {"X"=175347.79224858, "Y"=530230.992420933}, {"X"=175347.83379821095, "Y"=530231.0501731497}, {"X"=175347.87598747012, "Y"=530231.1085583183}, {"X"=175347.91865063147, "Y"=530231.1672461922}, {"X"=175347.96190239483, "Y"=530231.2254839465}, {"X"=175348.0049063384, "Y"=530231.2837890219}, {"X"=175348.04776506487, "Y"=530231.3412110822}, {"X"=175348.09002578325, "Y"=530231.3988968299}, {"X"=175348.1320544484, "Y"=530231.4565921396}, {"X"=175348.17388105046, "Y"=530231.5145510836}, {"X"=175348.2155488722, "Y"=530231.5718334815}, {"X"=175348.25715479362, "Y"=530231.6288519169}, {"X"=175348.298702659, "Y"=530231.6857062625}, {"X"=175348.34000642208, "Y"=530231.7423881912}, {"X"=175348.38131569765, "Y"=530231.7988370324}, {"X"=175348.42291422226, "Y"=530231.8557500527}, {"X"=175348.4651085602, "Y"=530231.9128555425}, {"X"=175348.5074611014, "Y"=530231.9701425808}, {"X"=175348.54977016072, "Y"=530232.0277038846}, {"X"=175348.59204602803, "Y"=530232.085123225}, {"X"=175348.63413675412, "Y"=530232.1425386709}, {"X"=175348.6759034338, "Y"=530232.200305787}, {"X"=175348.71787818449, "Y"=530232.2589446416}, {"X"=175348.76045198838, "Y"=530232.317371966}, {"X"=175348.80372661783, "Y"=530232.3755574945}, {"X"=175348.8467706997, "Y"=530232.4330600277}, {"X"=175348.88973412907, "Y"=530232.4902464917}, {"X"=175348.9325830176, "Y"=530232.5467385219}, {"X"=175348.97525145314, "Y"=530232.6036150943}, {"X"=175349.01743876605, "Y"=530232.6613454565}, {"X"=175349.05979153828, "Y"=530232.719614725}, {"X"=175349.1024098835, "Y"=530232.7775280537}, {"X"=175349.1453880101, "Y"=530232.8351950453}, {"X"=175349.18802687485, "Y"=530232.8922581619}, {"X"=175349.23083361104, "Y"=530232.9488757306}, {"X"=175349.2737960797, "Y"=530233.0057381197}, {"X"=175349.31699101478, "Y"=530233.0627330062}, {"X"=175349.35974836414, "Y"=530233.1203262894}, {"X"=175349.40281906206, "Y"=530233.1778453963}, {"X"=175349.44570093186, "Y"=530233.2353117875}, {"X"=175349.4887297444, "Y"=530233.2927455591}, {"X"=175349.53150355406, "Y"=530233.3505141508}, {"X"=175349.5747305128, "Y"=530233.4081582131}, {"X"=175349.61876782076, "Y"=530233.4660540435}, {"X"=175349.66334610982, "Y"=530233.5235709278}, {"X"=175349.70725425257, "Y"=530233.5815204117}, {"X"=175349.7504956164, "Y"=530233.639544004}, {"X"=175349.79353860093, "Y"=530233.6972796193}, {"X"=175349.83754390068, "Y"=530233.7539336112}, {"X"=175349.88171600256, "Y"=530233.8106814525}, {"X"=175349.92563081637, "Y"=530233.8675898704}, {"X"=175349.96906826223, "Y"=530233.9251234373}, {"X"=175350.01293208322, "Y"=530233.9821629709}, {"X"=175350.05650620023, "Y"=530234.0394841522}, {"X"=175350.09989550654, "Y"=530234.096613872}, {"X"=175350.14314725774, "Y"=530234.1536552103}, {"X"=175350.18660337463, "Y"=530234.2106127074}, {"X"=175350.2305396156, "Y"=530234.2675798872}, {"X"=175350.2749188809, "Y"=530234.3239919407}, {"X"=175350.31926038675, "Y"=530234.3805162015}, {"X"=175350.36325309795, "Y"=530234.4371080835}, {"X"=175350.40650135832, "Y"=530234.4938686392}, {"X"=175350.44973874703, "Y"=530234.5505470965}, {"X"=175350.49322314374, "Y"=530234.6074834237}, {"X"=175350.5372465261, "Y"=530234.6645657729}, {"X"=175350.58161553548, "Y"=530234.7214062652}, {"X"=175350.62636864078, "Y"=530234.7781335282}, {"X"=175350.67098936674, "Y"=530234.8347268899}, {"X"=175350.71522448817, "Y"=530234.8915222726}, {"X"=175350.75861984972, "Y"=530234.9483045933}, {"X"=175350.80163544806, "Y"=530235.0051679431}, {"X"=175350.8455027871, 
